vi "Parse Serial Number File.vi"(11 "String":string) -> (3 "Array":string[](array[string]))   [LabVIEW 2015]
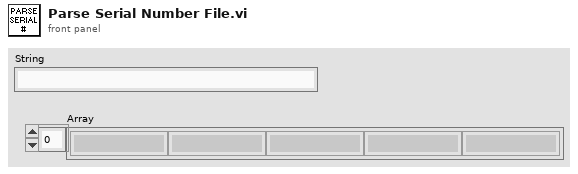
[diagram p1: front panel]
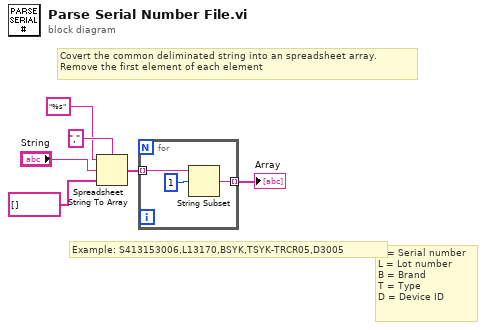
[diagram p0: block diagram]
diagram:
  # "S = Serial number\nL = Lot number\nB = Brand\nT = Type\nD = Device ID"
  # "Example: S413153006,L13170,BSYK,TSYK-TRCR05,D3005"
  # "Covert the common deliminated string into an spreadsheet array. \nRemove the first element of each element"
  n1 = Spreadsheet String To Array(delimiter (Tab)=",", format string="%s" ("spreadsheet string"), spreadsheet string="String", array type (2D Dbl)=string[] []) -> (array=w5:string[])
  n2 = for {
    tunnel: w5 -> [w9] mode=indexing
    tunnel: [w7] -> w6 mode=indexing
    n3 = String Subset(string=w9, offset (0)=1) -> (substring=w7:string)  [unwired: 1 in]
  }
  "Array" <- w6
